vi "Generate Library from TCF.vi"(0 "APG Config":T1={"APG Config"={"IPF Folder"=path "", "Results Folder"=path "", "Trace Folder"=path "", "a3DiCAD"={"Plot Spacing"=0.0, "TCF"=enum."STANDARD", "LeadLimit"=0, "a3DiCADDebug"=FALSE, "ODB"={"PrimePartNumber"=[], "SecondPartNumber"=[], "Height"={"PRP_CMP"="", "HEIGHT"=""}, "Units"={"PRP_CMP"="", "UNITS"=""}}, "PasteHeight"=0.0, "Inspection Performance"=TRUE}, "a3DiCADcfg"=path "", "Board Library"={"Board Library file"=path "", "Board library model folder"=path "", "Not Fittted/Fitted Components"=path "", "Panel Picture File"=path "", "Components"=enum."Fitted"}, "Site Library"={"Site Library file"=path "", "Site library model folder"=path ""}, "System Library"={"System Library file"=path "", "System library model folder"=path ""}, "ODB++ file"=path "", "Side ID Alias"={"Top"="", "Bottom"=""}}, "a3Di-cfg file"=path ""}, 5 "Inspection Data":T2, 11 "error in":errorcluster) -> (4 "APG Config":T1={"APG Config"={"IPF Folder"=path "", "Results Folder"=path "", "Trace Folder"=path "", "a3DiCAD"={"Plot Spacing"=0.0, "TCF"=enum."STANDARD", "LeadLimit"=0, "a3DiCADDebug"=FALSE, "ODB"={"PrimePartNumber"=[], "SecondPartNumber"=[], "Height"={"PRP_CMP"="", "HEIGHT"=""}, "Units"={"PRP_CMP"="", "UNITS"=""}}, "PasteHeight"=0.0, "Inspection Performance"=TRUE}, "a3DiCADcfg"=path "", "Board Library"={"Board Library file"=path "", "Board library model folder"=path "", "Not Fittted/Fitted Components"=path "", "Panel Picture File"=path "", "Components"=enum."Fitted"}, "Site Library"={"Site Library file"=path "", "Site library model folder"=path ""}, "System Library"={"System Library file"=path "", "System library model folder"=path ""}, "ODB++ file"=path "", "Side ID Alias"={"Top"="", "Bottom"=""}}, "a3Di-cfg file"=path ""}, 6 "Library successfully generated":bool, 8 "Library Generation cancelled":bool, 15 "error out":errorcluster)   [LabVIEW 2013, in "Manipulate IPF.lvlib"]
uses:
  Manipulate IPF.lvlib
  3013/code/Modules/GUI/GUI_5/subPanels/edit/type_def/data.ctl
  3013/code/Modules/Configuration/type_def/Scan Params.ctl
  3013/code/Modules/Configuration/type_def/Profile Resolution.ctl
  3013/code/Modules/Preprocess Data/type_def/direction.ctl
  3013/code/Modules/Inspection/Data/Panel_class/type_def/Config File data.ctl
  3013/code/Modules/Inspection/type_def/Pos and Rot.ctl
  3013/code/Modules/Inspection/Data/PCB_class/type_def/PCB Params.ctl
  3013/code/Modules/Inspection/Data/Panel_class/type_def/BarCode Params.ctl
  3013/code/Modules/Barcode Reader/type_def/id.ctl
  3013/code/Modules/Inspection/Data/Panel_class/type_def/inspection data.ctl
  3013/code/Modules/Inspection/type_def/Range Limits.ctl
  Settings/type_def/APG Config.ctl
  <userlib>/_OpenG.lib/file/file.llb/File Exists - Scalar__ogtk.vi
  Settings/Globals/apg_cfg_global.vi
  Mike/APG_mike a3Di.lvlib
  Settings/APG_settings.lvlib
  3013/code/Modules/Inspection/Inspection.lvlib
  3013/code/Modules/Inspection/Data/PCB_class/PCB.lvclass
  3013/code/Modules/Barcode Reader/Barcode Reader.lvlib
  3013/code/Modules/Inspection/Data/Panel_class/Panel.lvclass
  3013/code/Modules/Configuration/Config.lvlib
  3013/code/Modules/Preprocess Data/PreProcess.lvlib
  3013/code/Modules/GUI/GUI_5/subPanels/edit/edit.lvlib
panel:
  out "standard output":string
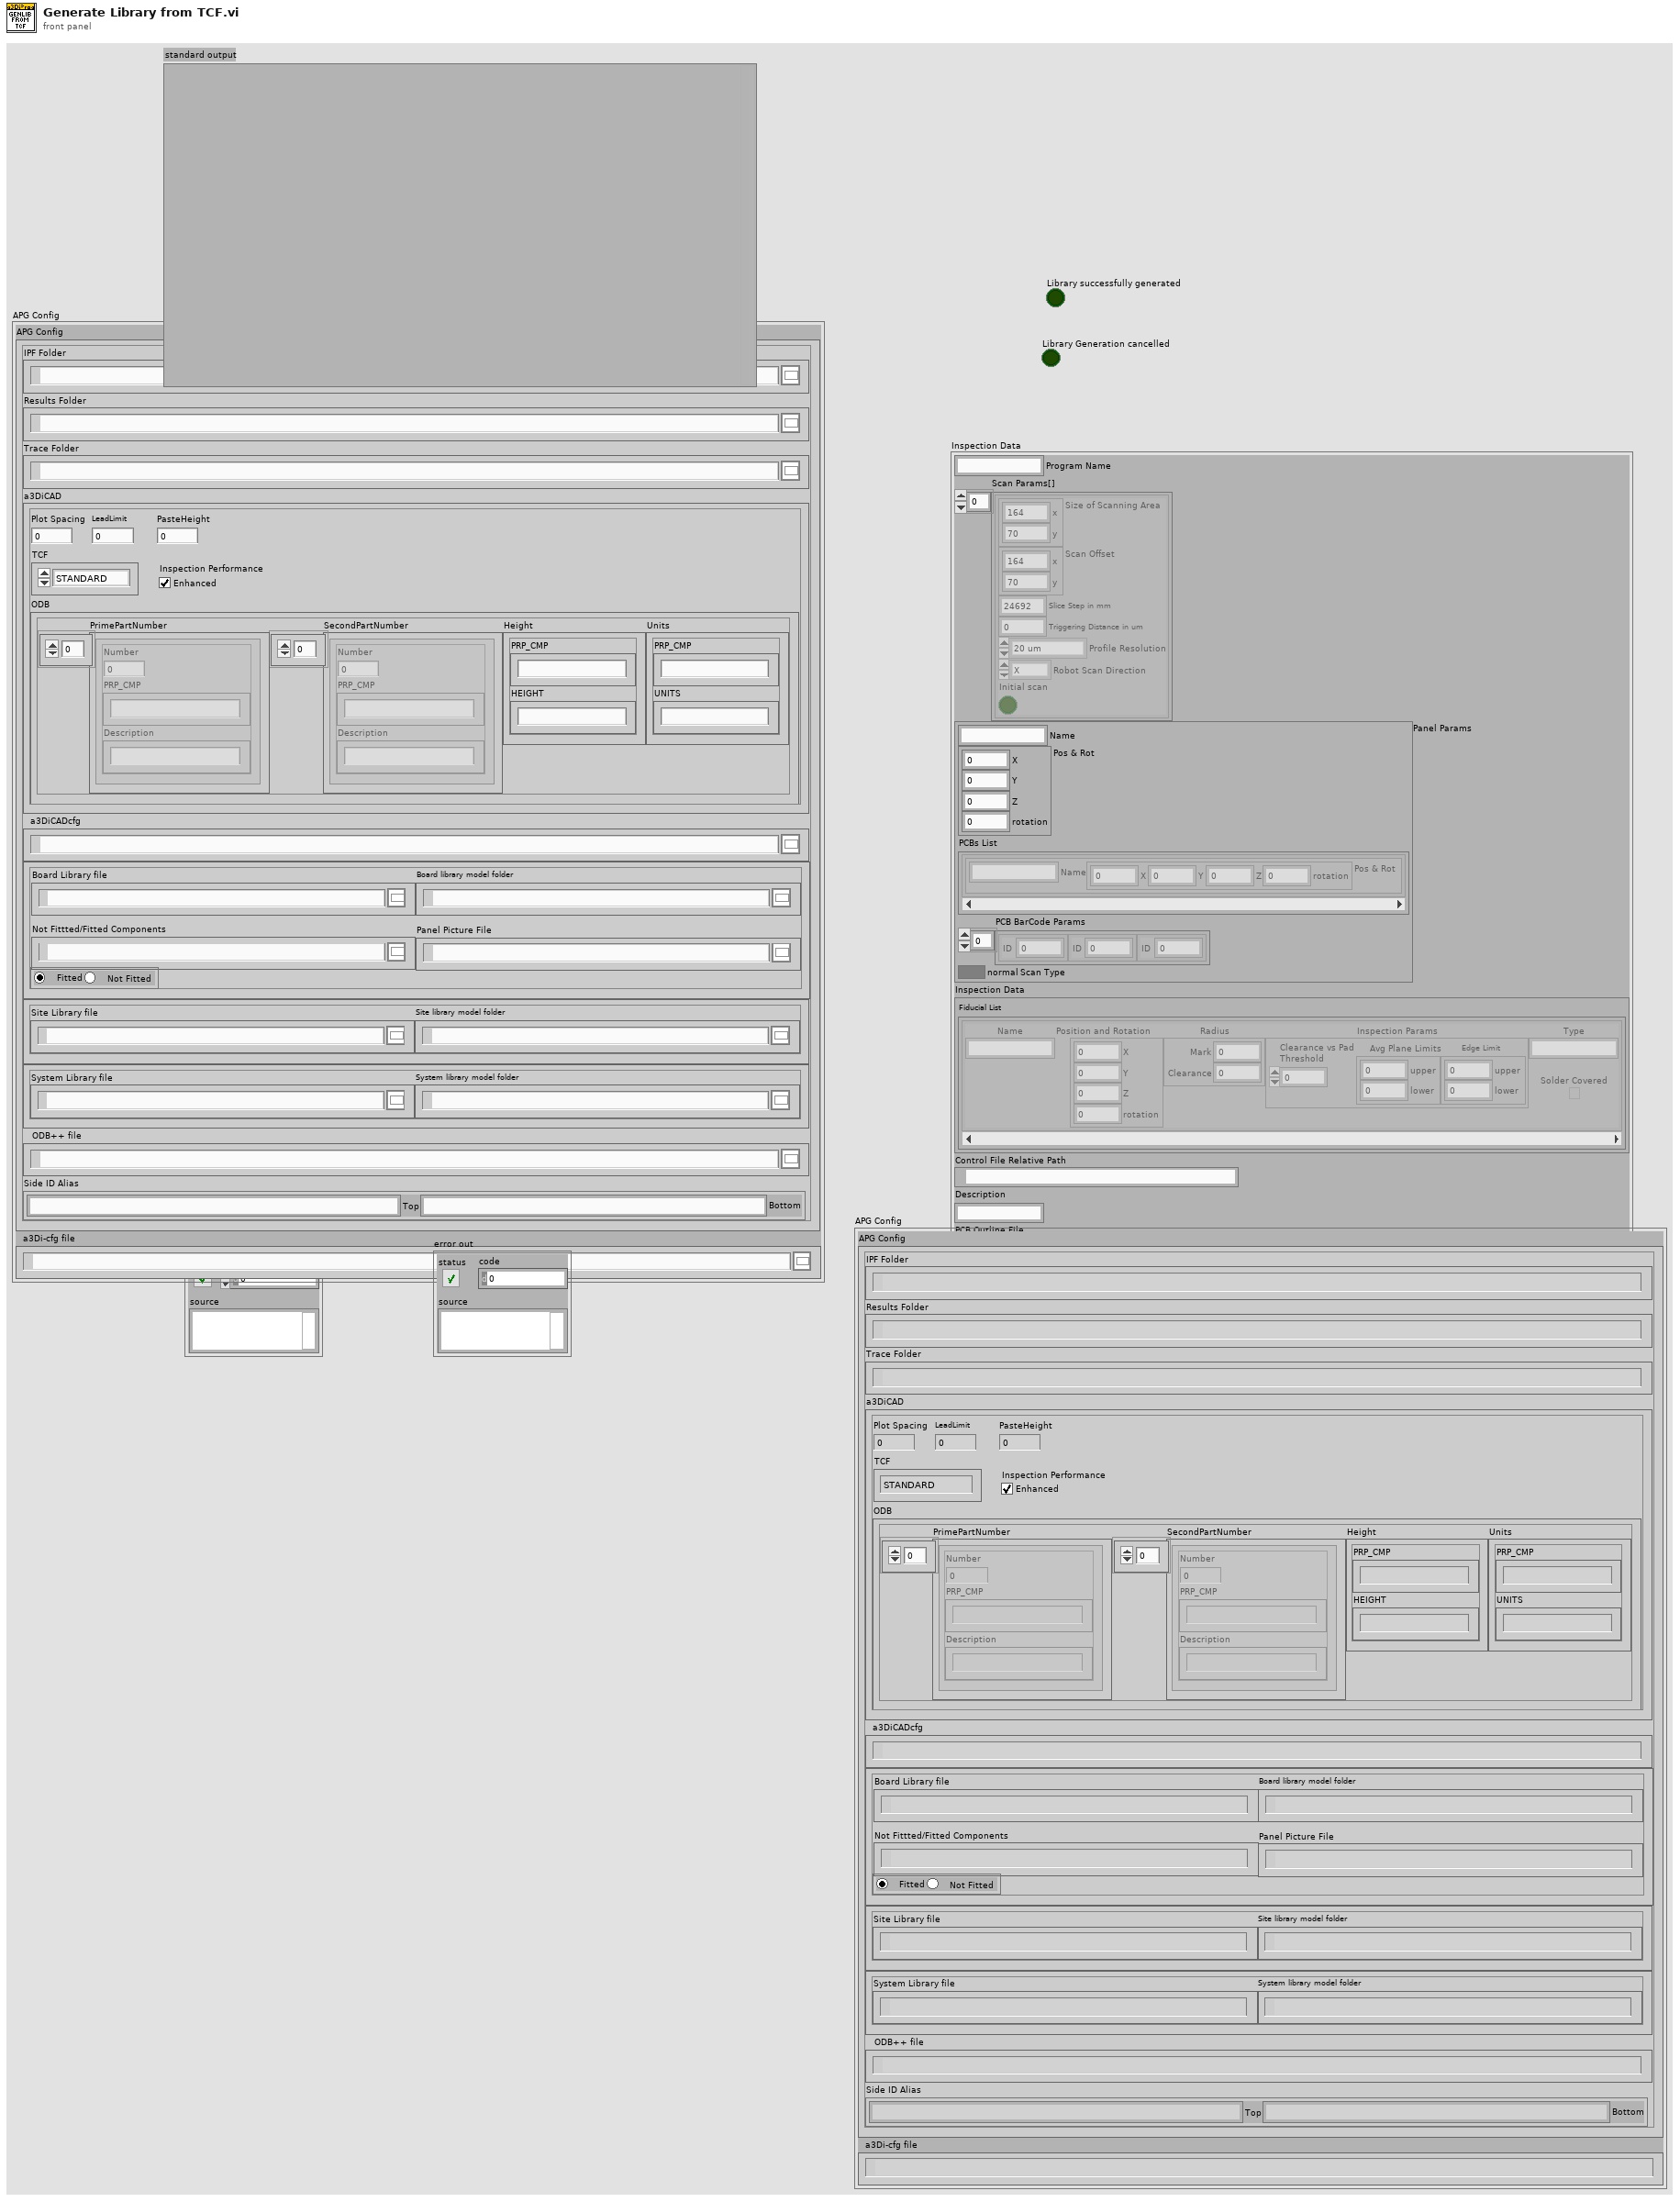
[diagram p1: front panel]
types:
  T1 = typedef "APG_settings.lvlib/APG Config.ctl" = cluster{"APG Config":cluster{"IPF Folder":path, "Results Folder":path, "Trace Folder":path, "a3DiCAD":cluster{"Plot Spacing":dbl, "TCF":enum16{"STANDARD", "PASTE", "LEAD"}, "LeadLimit":u32, "a3DiCADDebug":bool, "ODB":cluster{"PrimePartNumber":cluster{"Number":u32, "PRP_CMP":string, "Description":string}[], "SecondPartNumber":cluster{"Number":u32, "PRP_CMP":string, "Description":string}[], "Height":cluster{"PRP_CMP":string, "HEIGHT":string}, "Units":cluster{"PRP_CMP":string, "UNITS":string}}, "PasteHeight":dbl, "Inspection Performance":bool}, "a3DiCADcfg":path, "Board Library":cluster{"Board Library file":path, "Board library model folder":path, "Not Fittted/Fitted Components":path, "Panel Picture File":path, "Components":enum32{"Fitted", "Not Fitted "}}, "Site Library":cluster{"Site Library file":path, "Site library model folder":path}, "System Library":cluster{"System Library file":path, "System library model folder":path}, "ODB++ file":path, "Side ID Alias":cluster{"Top":string, "Bottom":string}}, "a3Di-cfg file":path}
  T2 = typedef "GUI.lvlib/subPanel.lvlib/edit.lvlib/data.ctl" = cluster{"Program Name":string, "Scan Params[]":T3[], "Panel Params":T6, "Inspection Data":T11, "Control File Relative Path":path, "Description":string, "PCB Outline File":path, "Scan Start Delay":dbl, "CAD Picture File":string, "Product Code":string, "Side ID":string}
  T3 = typedef "Config.lvlib/Scan Params.ctl" = cluster{"Size of Scanning Area":cluster{"x":dbl, "y":dbl}, "Scan Offset":cluster{"x":dbl, "y":dbl}, "Slice Step in mm":dbl, "Triggering Distance in mm":dbl, "Triggering Distance in um":dbl, "Profile Resolution":T4, "Version":string, "Robot Scan Direction":T5, "Initial scan":bool}
  T4 = typedef "Config.lvlib/Profile Resolution.ctl" = enum8{"20 um", "40 um"}
  T5 = typedef "PreProcess.lvlib/direction.ctl" = enum8{"X", "Y"}
  T6 = typedef "Inspection.lvlib/Panel.lvclass/Config File data.ctl" = cluster{"Name":string, "Pos & Rot":T7, "PCBs List":cluster{"PCB Params":T8}[], "PCB BarCode Params":T9[], "Scan Type":bool}
  T7 = typedef "Inspection.lvlib/Pos and Rot.ctl" = cluster{"X":dbl, "Y":dbl, "Z":dbl, "rotation":dbl}
  T8 = typedef "Inspection.lvlib/PCB.lvclass/PCB Params.ctl" = cluster{"Name":string, "Pos & Rot":T7}
  T9 = typedef "Inspection.lvlib/Panel.lvclass/BarCode Params.ctl" = cluster{"ID":T10}
  T10 = typedef "Barcode Reader.lvlib/id.ctl" = u8
  T11 = typedef "Inspection.lvlib/Panel.lvclass/inspection data.ctl" = cluster{"Fiducial List":cluster{"Name":string, "Position and Rotation":T7, "Radius":cluster{"Mark":dbl, "Clearance":dbl}, "Inspection Params":cluster{"Clearance vs Pad\nThreshold":dbl, "Avg Plane Limits":T12, "Edge Limit":T12}, "Type":string, "Solder Covered":bool}[]}
  T12 = typedef "Inspection.lvlib/Range Limits.ctl" = cluster{"upper":sgl, "lower":sgl}
  T13 = cluster{"ODB2CPF.exe":path, "TCFToArtworkCPF.exe":path, "TCFToCPFLabels.exe":path, "7z.exe":path, "UpdateTCFLibrary.exe":path, "a3DiPackageTests":path, "Error Codes":path, "TCFToCuboidRefCPF":path, "TCFToArtworkRefCPF":path, "ExtractPKG":path, "ExtractTCFFromODBFileForPKG":path, "OutLineFilterTCFPKG":path, "GenerateLibraryFromTCF":path, "FlipCPF":path, "FlipTCF":path, "TCFToJointBridgeCPF":path, "TCFToJointFR4CPF":path, "UpdateTCFPartNoFrCompName":path}
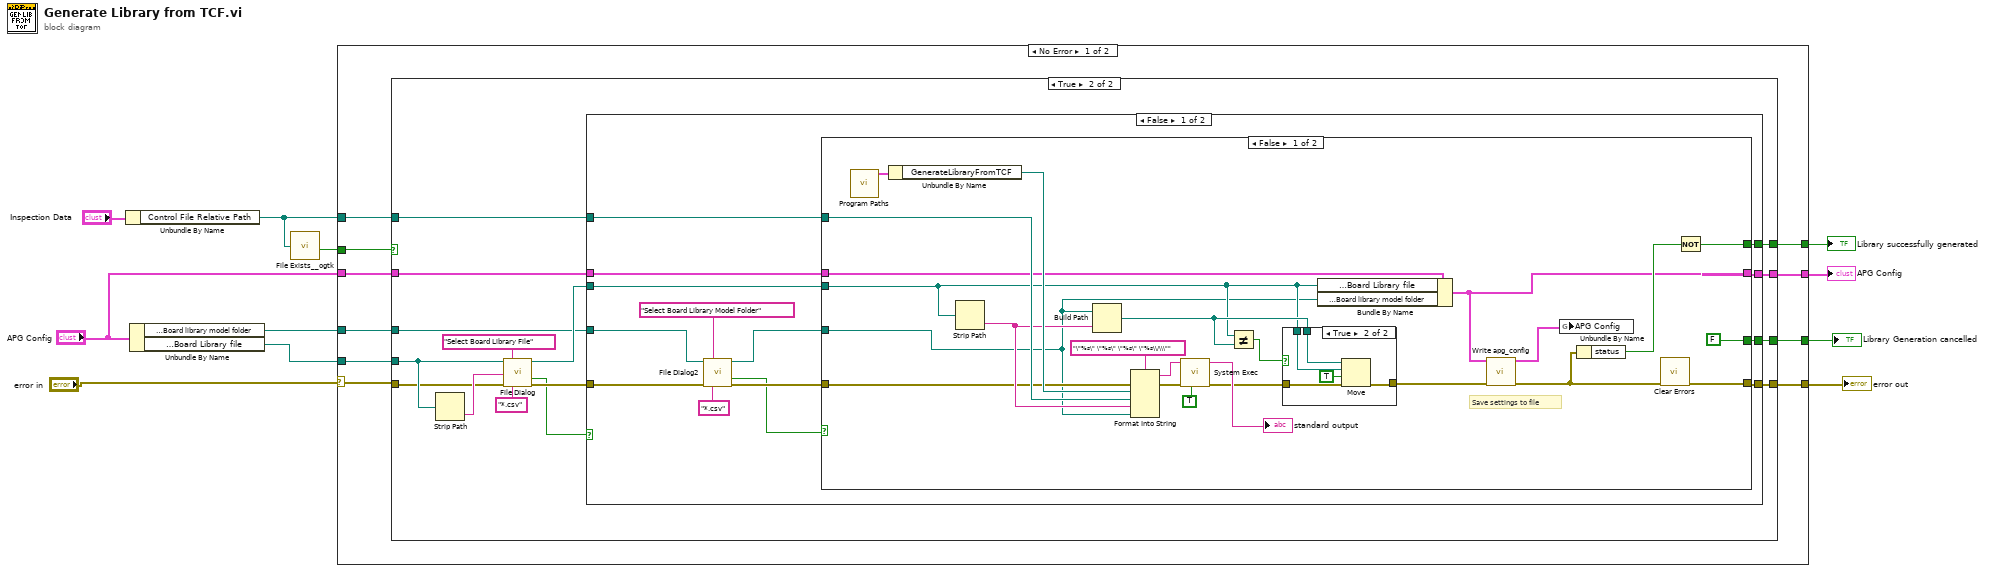
[diagram p0: block diagram]
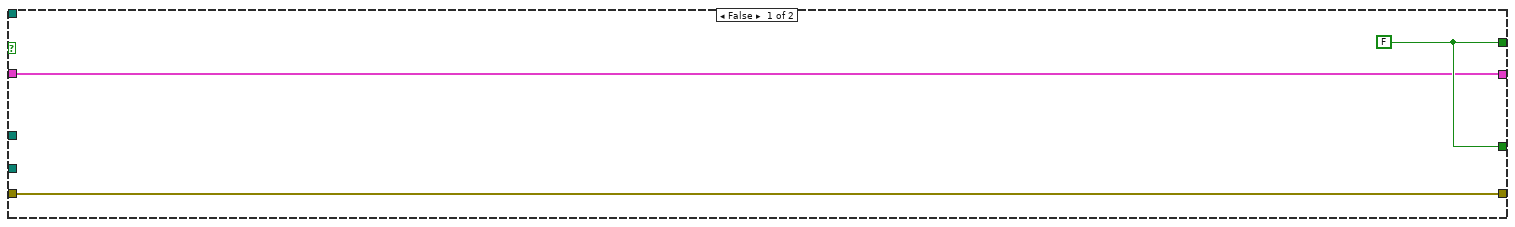
[diagram p2: hidden frame]
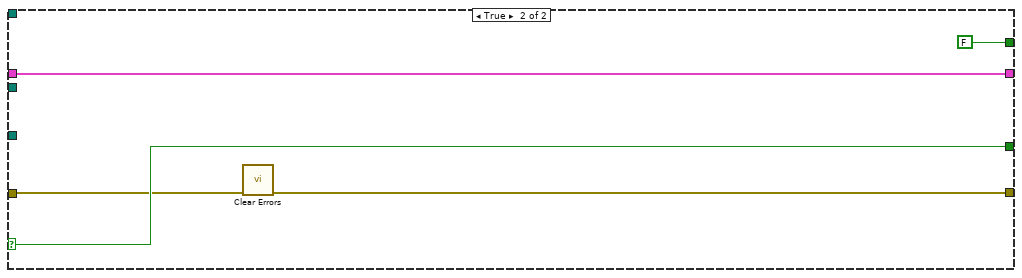
[diagram p4: hidden frame]
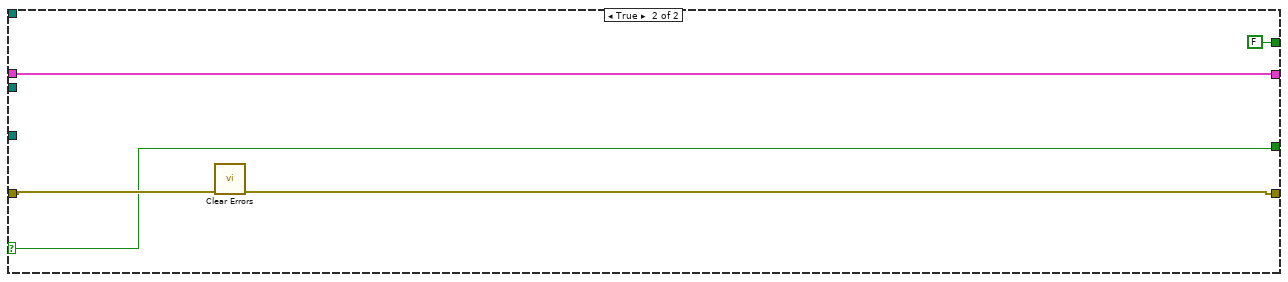
[diagram p5: hidden frame]
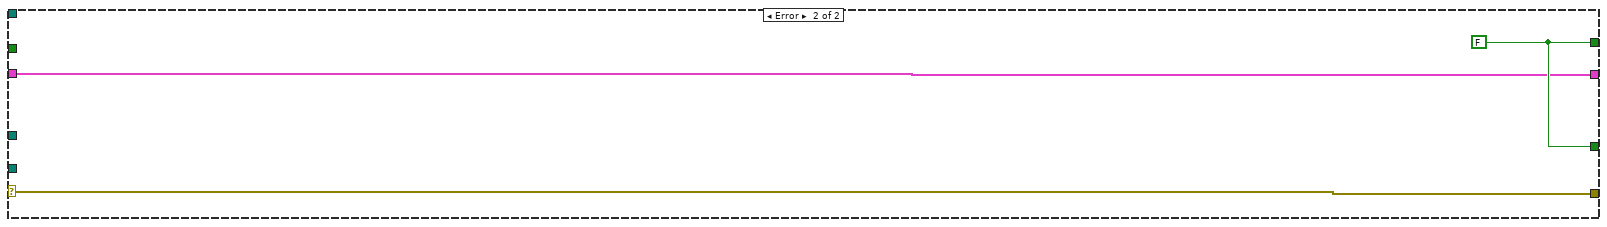
[diagram p6: hidden frame]
diagram:
  n1 = Unbundle By Name("Inspection Data") -> ("Control File Relative Path"=w8:path)
  n2 = Unbundle By Name("APG Config") -> ("APG Config.Board Library.Board library model folder"=w5:path, "APG Config.Board Library.Board Library file"=w4:path)
  n3 = call-poly <userlib>:"File Exists__ogtk.vi"("file path"=w8) -> ("exists"=w10:bool)  [unwired: 6 in, 1 out]
  n4 = case shown="No Error" "error in" {
    selector: "error in" -> [w17 w96]
    tunnel: w10 -> [w21 _]
    tunnel: [w20 w96] -> w9
    tunnel: w8 -> [w19 _]
    tunnel: [w18 w95] -> w7
    tunnel: w5 -> [w16 _]
    tunnel: w4 -> [w15 _]
    tunnel: [w14 w95] -> w3
    tunnel: "APG Config" -> [w13 w94]
    tunnel: [w12 w94] -> w1
    frame No Error {
      n5 = case shown="True" w21 {
        tunnel: w19 -> [_ w39]
        tunnel: w17 -> [w24 w29]
        tunnel: [w24 w35] -> w20
        tunnel: [w23 w38] -> w18
        tunnel: w16 -> [_ w26]
        tunnel: w15 -> [_ w30]
        tunnel: [w23 w36] -> w14
        tunnel: w13 -> [w22 w32]
        tunnel: [w22 w31] -> w12
        frame False {
          w23 = FALSE
        }
        frame True {
          n6 = Strip Path(path=w30) -> (name=w34:string)  [unwired: 1 out]
          n7 = call "File Dialog"("start path"=w30, "prompt"="Select Board Library File", "default name"=w34, "error in"=w29, "pattern (all files)"="*.csv") -> ("selected path"=w28:path, "cancelled"=w25:bool, "error out"=w27:errorcluster)  [unwired: 7 in, 1 out]
          n8 = case shown="False" w25 {
            selector: w25 -> [_ w91]
            tunnel: w39 -> [w53 _]
            tunnel: [w52 FALSE] -> w38
            tunnel: [w51 w91] -> w36
            tunnel: [w50 w92] -> w35
            tunnel: w32 -> [w49 w89]
            tunnel: [w48 w89] -> w31
            tunnel: w28 -> [w46 _]
            tunnel: w27 -> [w45 w93]
            tunnel: w26 -> [w41 _]
            frame False {
              n9 = call "File Dialog2"("start path"=w41, "prompt"="Select Board Library Model Folder", "error in"=w45, "pattern (all files)"="*.csv") -> ("selected path"=w43:path, "cancelled"=w40:bool, "error out"=w44:errorcluster)  [unwired: 8 in, 1 out]
              n10 = case shown="False" w40 {
                selector: w40 -> [_ w88]
                tunnel: w53 -> [w72 _]
                tunnel: [w66 FALSE] -> w52
                tunnel: w44 -> [w62 w86]
                tunnel: w43 -> [w58 _]
                tunnel: [FALSE w88] -> w51
                tunnel: [w61 w85] -> w50
                tunnel: w49 -> [w60 w84]
                tunnel: [w54 w84] -> w48
                tunnel: w46 -> [w59 _]
                frame False {
                  # "Save settings to file"
                  n11 = call "Program Paths.vi"() -> ("Program paths"=w73:T13)  [unwired: 10 in]
                  n12 = Unbundle By Name(w73) -> ("GenerateLibraryFromTCF"=w70:path)
                  n13 = Strip Path(path=w59) -> (name=w68:string)  [unwired: 1 out]
                  n14 = Build Path(base path=w58, name or relative path=w68) -> (appended path=w65:path)
                  n15 = Format Into String(format string="\"%s\" \"%s\" \"%s\" \"%s\\/\\\"", error in=w62, w70, w72, w68, w58) -> (resulting string=w77:string, error out=w75:errorcluster)  [unwired: 1 in]
                  n16 = call <vilib>:"System Exec.vi"("run minimized? (F)"=TRUE, "error in (no error)"=w75, "command line"=w77) -> ("error out"=w69:errorcluster, "standard output"=→"standard output":string)  [unwired: 5 in, 2 out]
                  n17 = Not Equal?(x=w59, y=w65) -> (x != y?=w64:bool)
                  n18 = case shown="True" w64 {
                    tunnel: w69 -> [w78 w83]
                    tunnel: [w78 w81] -> w55
                    tunnel: w59 -> [_ w80]
                    tunnel: w65 -> [_ w79]
                    frame False {
                    }
                    frame True {
                      n19 = Move(source path=w79, error in=w83, 9:TRUE ("overwrite (F)"), 10:w80) -> (error out=w81:errorcluster)  [unwired: 1 in, 2 out]
                    }
                  }
                  n20 = Bundle By Name(cluster=w60, "APG Config.Board Library.Board Library file"=w59, "APG Config.Board Library.Board library model folder"=w58) -> (w54:T1)
                  n21 = call "Write apg_config.vi"("APG Config"=w54, "error in (no error)"=w55) -> ("APG Config out"=w57:T1, "error out"=w56:errorcluster)  [unwired: 12 in]
                  n22 = global write "apg_cfg_global.vi" "APG Config"(w57) -> ()
                  n23 = Unbundle By Name(w56) -> ("status"=w67:bool)
                  n24 = call <vilib>:"Clear Errors.vi"("error in (no error)"=w56) -> ("error out"=w61:errorcluster)  [unwired: 6 in]
                  n25 = Not(x=w67) -> (.not. x?=w66:bool)
                }
                frame True {
                  n26 = call <vilib>:"Clear Errors.vi"("error in (no error)"=w86) -> ("error out"=w85:errorcluster)  [unwired: 6 in]
                }
              }
            }
            frame True {
              n27 = call <vilib>:"Clear Errors.vi"("error in (no error)"=w93) -> ("error out"=w92:errorcluster)  [unwired: 6 in]
            }
          }
        }
      }
    }
    frame Error {
      w95 = FALSE
    }
  }
  "error out" <- w9
  "Library successfully generated" <- w7
  "Library Generation cancelled" <- w3
  "APG Config" <- w1
